vi "Get Components.vi"(8 "error in (no error)":errorcluster, 11 "Plugin Configuration in":refnum<class "Plugin Configuration.lvclass">) -> (0 "error out":errorcluster, 2 "components":string[](array[string]), 3 "Plugin Configuration out":refnum<class "Plugin Configuration.lvclass">)   [LabVIEW 2021, in "DSF Core.lvlib" / "Plugin Configuration.lvclass"]
uses:
  Plugin Configuration.lvclass
  Plugin Configuration.lvclass/Plugin Configuration.ctl
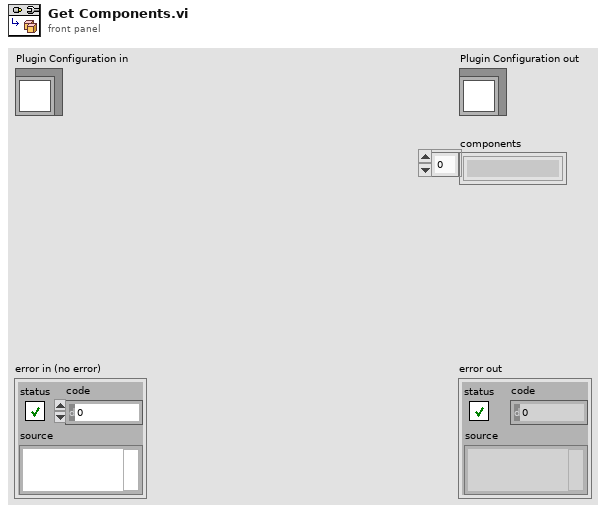
[diagram p1: front panel]
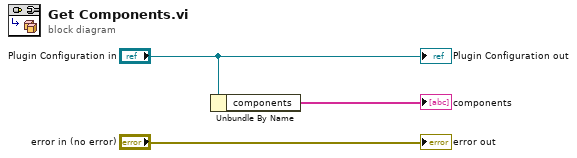
[diagram p0: block diagram]
diagram:
  n1 = Unbundle By Name("Plugin Configuration in") -> ("components"=→"components":string[])
  "error out" <- "error in (no error)"
  "Plugin Configuration out" <- "Plugin Configuration in"
